vi "TimeFGV.vi"(2 "TimeFGV상태":enum16{"초기화", "카운팅"}(ring), 3 "목표시간":dbl) -> (0 "현재 시간":dbl, 1 "도달?":bool)   [LabVIEW 2020]
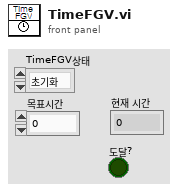
[diagram p1: front panel]
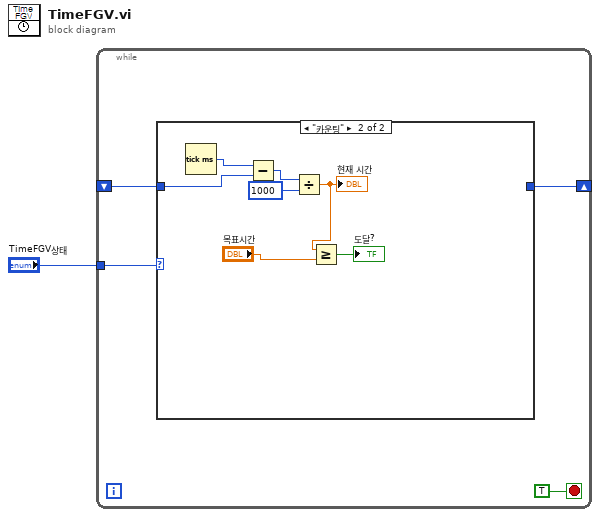
[diagram p0: block diagram]
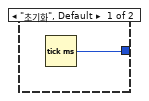
[diagram p2: hidden frame]
diagram:
  n1 = while {
    tunnel: "TimeFGV상태" -> [w4]
    shift-right: [w3] -> _
    shift-left: _ -> [w2]
    stop <- TRUE stop-if-true
    n2 = case shown="\"카운팅\"" w4 {
      tunnel: [w6 _] -> w3
      tunnel: w2 -> [_ w11]
      frame "초기화", Default {
        n3 = Tick Count (ms)() -> (millisecond timer value=w6:u32)
      }
      frame "카운팅" {
        n4 = Tick Count (ms)() -> (millisecond timer value=w12:u32)
        n5 = Subtract(x=w12, y=w11) -> (x-y=w13:u32)
        n6 = Divide(x=w13, y=u32 1000) -> (x/y=w8:dbl)
        "현재 시간" <- w8
        n7 = Greater Or Equal?(x=w8, y="목표시간") -> (x >= y?=→"도달?":bool)
      }
    }
  }
